vi "0xEE_Cmd_read_device_description_fragment_in_JSON_format_(SubVI).vi"(8 "error in":errorcluster, 9 "Смешение в байтах":i32, 10 "Макс размер":i32, 11 "String in":string) -> (0 "error out":errorcluster, 3 "String out":string)   [LabVIEW 2017, in "LV_Unicorn.lvlib"]
uses:
  LV_Unicorn.lvlib
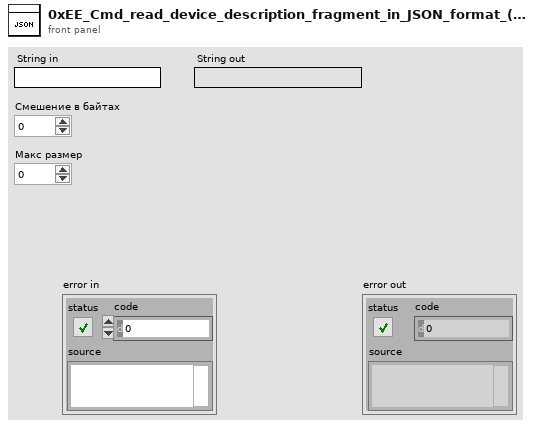
[diagram p1: front panel]
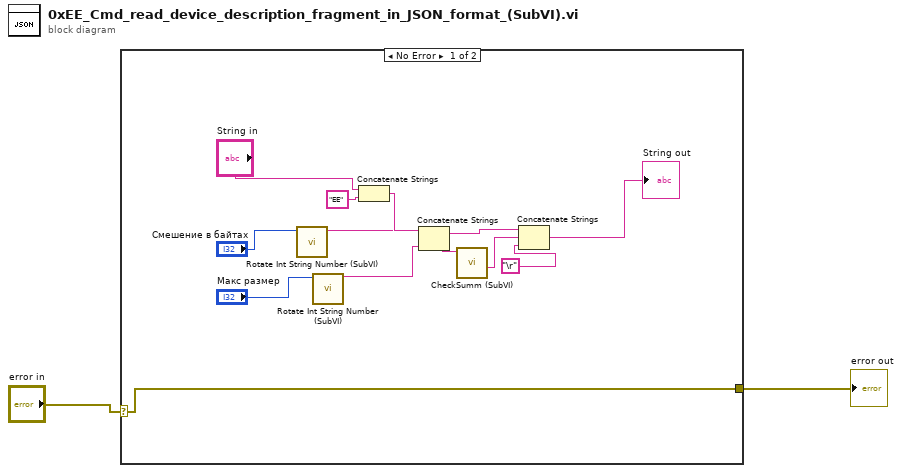
[diagram p0: block diagram]
diagram:
  n1 = case shown="No Error" "error in" {
    selector: "error in" -> [w3 w15]
    tunnel: [w3 w15] -> w1
    frame No Error {
      n2 = call "Rotate Int String Number (SubVI).vi"("Int Number In"="Смешение в байтах") -> ("Orig String"=w6:string)  [unwired: 8 in, 2 out]
      n3 = call "Rotate Int String Number (SubVI).vi"("Int Number In"="Макс размер") -> ("Orig String"=w7:string)  [unwired: 8 in, 2 out]
      n4 = Concatenate Strings("String in", "EE" ("string")) -> (w12:string)
      n5 = Concatenate Strings(w12, w6, w7) -> (w9:string)
      n6 = call "CheckSumm (SubVI).vi"("Input String"=w9) -> ("CheckSumm"=w8:string)  [unwired: 7 in, 3 out]
      n7 = Concatenate Strings(w9, w8, "\r") -> (→"String out":string)
    }
    frame Error {
    }
  }
  "error out" <- w1
